vi "Untitled 17.vi"   [LabVIEW 2020]
uses:
  Multimetro/Multimetro.lvclass
  Instrumento feo/Instrumento feo.lvclass
  D:/Storage/Source Code/Clase AF/ClaseAF/11 OOP Interfaces/Instrumento/Instrumento.lvclass
  D:/Storage/Source Code/Clase AF/ClaseAF/11 OOP Interfaces/Multimetro/Multimetro.lvclass
  D:/Storage/Source Code/Clase AF/ClaseAF/11 OOP Interfaces/Mediciones/Mediciones.lvclass
  D:/Storage/Source Code/Clase AF/ClaseAF/11 OOP Interfaces/Instrumento feo/Instrumento feo.lvclass
  Mediciones/Mediciones.lvclass
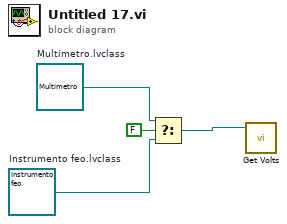
[diagram p0: block diagram]
diagram:
  w2 = refnum<class "Instrumento feo.lvclass"> refnum  # Instrumento feo.lvclass
  w4 = refnum<class "Multimetro.lvclass"> refnum  # Multimetro.lvclass
  n1 = Select(t=w4, s=FALSE, f=w2) -> (s? t:f=w3:refnum<class "Mediciones.lvclass">)
  n2 = call-dynamic "Get Volts.vi"("Mediciones in"=w3) -> ()  [unwired: 8 in, 3 out]
